vi "20220303-001 test.vi"() -> ()   [LabVIEW 2019]
uses:
  subVI/move/position cluster.ctl
  52/sub/route_name.ctl
panel:
  out "error out":errorcluster
  in  "error in (no error)":errorcluster
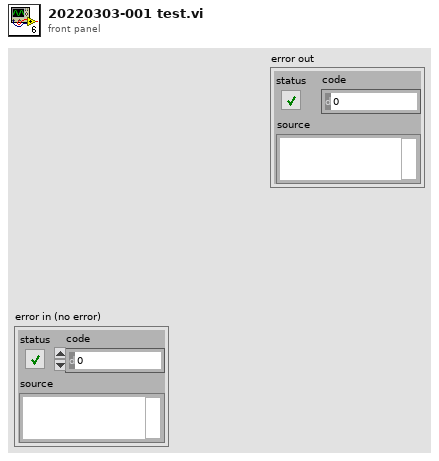
[diagram p1: front panel]
types:
  T1 = typedef "route_name.ctl" = enum16{"S-Vision", "Vision-R1", "Vision-R2", "Vision-R3", "Vision-R4", "Vision-R5", "R1-Vision", "R2-Vision", "R3-Vision", "R4-Vision", "R5-Vision", "Vision-box", "box-recycle", "recycle-box", "box-Vision", "Vision-S"}
  T2 = typedef "position cluster.ctl" = cluster{"X":dbl, "Y":dbl, "Angle":dbl}
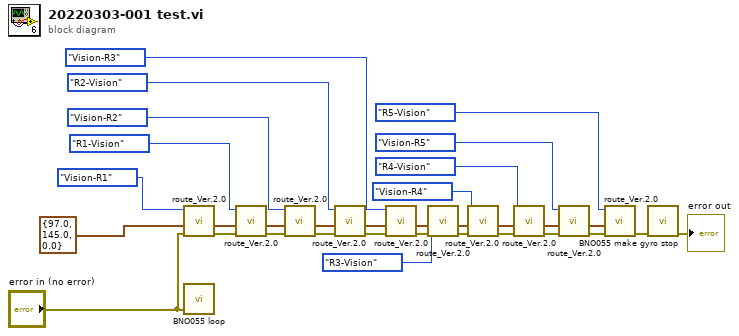
[diagram p0: block diagram]
diagram:
  n1 = call "route_Ver.2.0.vi"("error in (no error)"="error in (no error)", "Position"=T2 {"X"=97.0, "Y"=145.0, "Angle"=0.0}, 11:route_name."Vision-R1") -> ("error out"=w29:errorcluster, "Position out"=w28:T2)  [unwired: 7 in]
  n2 = call "BNO055 loop.vi"("error in (no error)"="error in (no error)") -> ()  [unwired: 11 in]
  n3 = call "route_Ver.2.0.vi"("error in (no error)"=w29, "Position"=w28, 11:route_name."R1-Vision") -> ("error out"=w27:errorcluster, "Position out"=w26:T2)  [unwired: 7 in]
  n4 = call "route_Ver.2.0.vi"("error in (no error)"=w27, "Position"=w26, 11:route_name."Vision-R2") -> ("error out"=w25:errorcluster, "Position out"=w24:T2)  [unwired: 7 in]
  n5 = call "route_Ver.2.0.vi"("error in (no error)"=w25, "Position"=w24, 11:route_name."R2-Vision") -> ("error out"=w8:errorcluster, "Position out"=w9:T2)  [unwired: 7 in]
  n6 = call "route_Ver.2.0.vi"("error in (no error)"=w8, "Position"=w9, 11:route_name."Vision-R3") -> ("error out"=w23:errorcluster, "Position out"=w22:T2)  [unwired: 7 in]
  n7 = call "route_Ver.2.0.vi"("error in (no error)"=w23, "Position"=w22, 11:route_name."R3-Vision") -> ("error out"=w18:errorcluster, "Position out"=w19:T2)  [unwired: 7 in]
  n8 = call "route_Ver.2.0.vi"("error in (no error)"=w18, "Position"=w19, 11:route_name."Vision-R4") -> ("error out"=w21:errorcluster, "Position out"=w20:T2)  [unwired: 7 in]
  n9 = call "route_Ver.2.0.vi"("error in (no error)"=w21, "Position"=w20, 11:route_name."R4-Vision") -> ("error out"=w17:errorcluster, "Position out"=w16:T2)  [unwired: 7 in]
  n10 = call "route_Ver.2.0.vi"("error in (no error)"=w17, "Position"=w16, 11:route_name."Vision-R5") -> ("error out"=w15:errorcluster, "Position out"=w14:T2)  [unwired: 7 in]
  n11 = call "route_Ver.2.0.vi"("error in (no error)"=w15, "Position"=w14, 11:route_name."R5-Vision") -> ("error out"=w2:errorcluster)  [unwired: 7 in, 1 out]
  n12 = call "BNO055 make gyro stop .vi"("error in (no error)"=w2) -> ("error out"=→"error out":errorcluster)  [unwired: 10 in]
